vi "List.vi"(8 "error in (no error)":errorcluster, 11 "LUnit Test Suite In":refnum<class "LUnit Test Suite.lvclass">) -> (0 "error out":errorcluster, 2 "List of Runnables":string[](array[string]))   [LabVIEW 2020, in "LUnit Test Suite.lvclass"]
doc: "List all tests in suite."
uses:
  LUnit Test Suite.lvclass
  LUnit Test Suite.lvclass/LUnit Test Suite.ctl
  Runnable.lvclass
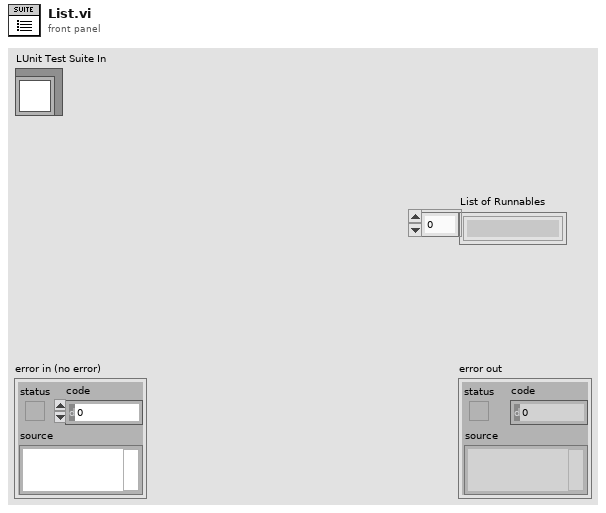
[diagram p1: front panel]
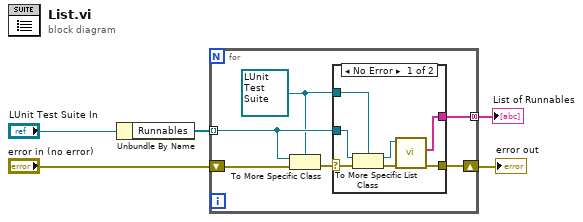
[diagram p0: block diagram]
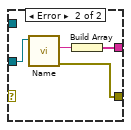
[diagram p2: hidden frame]
diagram:
  n1 = Unbundle By Name("LUnit Test Suite In") -> ("Runnables"=w4:refnum<class "Runnable.lvclass">[])
  n2 = for {
    tunnel: w4 -> [w11] mode=indexing
    tunnel: [w10] -> w3 mode=concatenating
    shift-right: [w8] -> w1
    shift-left: "error in (no error)" -> [w9]
    w6 = refnum<class "LUnit Test Suite.lvclass"> refnum ("LUnit Test Suite.lvclass")
    n3 = To More Specific Class(target class=w6, reference=w11, error in=w9) -> (error out=w7:errorcluster)  [unwired: 1 out]
    n4 = case shown="No Error" w7 {
      selector: w7 -> [w14 _]
      tunnel: [w18 w20] -> w10
      tunnel: [w17 w19] -> w8
      tunnel: w11 -> [w16 w22]
      tunnel: w6 -> [w15 _]
      frame No Error {
        n5 = To More Specific Class(target class=w15, reference=w16, error in=w14) -> (specific class reference=w12:refnum<class "LUnit Test Suite.lvclass">, error out=w13:errorcluster)
        n6 = call "List.vi"("error in (no error)"=w13, "LUnit Test Suite In"=w12) -> ("error out"=w17:errorcluster, "List of Runnables"=w18:string[])  [unwired: 8 in]
      }
      frame Error {
        n7 = call-dynamic "Name.vi"("Runnable in"=w22) -> ("error out"=w19:errorcluster, "Name"=w21:string)  [unwired: 8 in, 1 out]
        n8 = Build Array(w21) -> (w20:string[])
      }
    }
  }
  "error out" <- w1
  "List of Runnables" <- w3
